vi "SpamDigit_v13.vi"() -> ()   [LabVIEW 2015]
uses:
  <vilib>/Platform/TimedLoop/XDataNode/timing_clust.ctl
  <vilib>/Platform/TimedLoop/XDataNode/nitl_modes.ctl
  <vilib>/Platform/TimedLoop/XDataNode/wakeup.ctl
  <vilib>/Utility/inputDevices.llb/keyboardAcquire.vi
  <vilib>/Utility/file.llb/Write To Spreadsheet File (string).vi
  <vilib>/Platform/TimedLoop/XDataNode/XDataNode.xnode
  <vilib>/Platform/TimedLoop/XDataNode/XDNodeRunTimeDep.lvlib
panel:
  out "Spam 2":i32
  out "seg":bool
  out "prim":bool
  out "tempo_rel":dbl[](array[numeric])
  out "erro":dbl[](array[numeric])
  out "total":dbl[](array[numeric])
  in  "Tab Control":enum32{"Config", "Exec"}(tab)
  in  "msg_inver":string="Na tela irão aparecer uma sequência de números. Após a sequência a mensagem \"comece!\" aparecerá e imediatamente você deve digitar os números na ordem inversas que eles apareceram. A quantidade de números irá aumentar gradualmente.                                           Pressione a tecla \"0\" para iniciar!"
  in  "Spam_1_I":string="24"
  in  "Spam_2_I":string="415" caption="Spam_2"
  in  "Spam_1_2_I":string="57"
  in  "Spam_2_2_I":string="629"
  in  "Spam_3_I":string="3272" caption="Spam_2"
  in  "Spam_4_I":string="15286" caption="Spam_2"
  in  "Spam_5_I":string="539418" caption="Spam_2"
  in  "Spam_6_I":string="8129365" caption="Spam_2"
  in  "Spam_7_I":string="72819653" caption="Spam_2"
  in  "Spam_8_I":string="591742817" caption="Spam_2"
  in  "Spam_9_I":string="4273164395" caption="Spam_2"
  in  "Spam_3_2_I":string="4968"
  in  "Spam_4_2_I":string="61843"
  in  "Spam_5_3_I":string="724856"
  in  "Spam_6_2_I":string="4739128"
  in  "Spam_7_2_I":string="94376258"
  in  "Spam_8_2_I":string="417938663"
  in  "Spam_9_2_I":string="7583672861"
  in  "Spam_1":string="17"
  in  "N_max spam":i32=9
  in  "Spam_2":string="582"
  in  "Spam_1_2":string="63"
  in  "Spam_2_2":string="694"
  in  "sensib":i32=200
  in  "Tempo1":u32=500
  in  "Tempo_2":u32=500
  in  "Spam_3":string="6439" caption="Spam_2"
  in  "Spam_4":string="42731" caption="Spam_2"
  in  "Spam_5":string="619473" caption="Spam_2"
  in  "Spam_6":string="5917428" caption="Spam_2"
  in  "Spam_7":string="38295174" caption="Spam_2"
  in  "Spam_8":string="275862584" caption="Spam_2"
  in  "Spam_9":string="4739128415" caption="Spam_2"
  in  "Spam_3_2":string="7286"
  in  "Spam_4_2":string="75836"
  in  "Spam_5_2":string="619473"
  in  "Spam_6_2":string="4179386"
  in  "Spam_7_2":string="58192647"
  in  "Spam_8_2":string="713942568"
  in  "Spam_9_2":string="8129365629"
  in  "comece":i32=300
  in  "aguarde":i32=1000
  in  "msg_direto":string=" Na tela irão aparecer uma sequência de números. Após a sequência a mensagem \"comece!\" aparecerá e imediatamente você deve digitar os números na mesma ordem que eles apareceram. A quantidade de números irá aumentar gradualmente.                                            Pressione a tecla \"0\" para iniciar!"
  in  "direto":bool
  in  "inver":bool
  in  "ambos":bool
  in  "print":string
  out "Aguarde":string
  in  "iniciar":bool
  out "Comece":string
  out "msg":string
  out "array2":T1(array[ring])
  in  "Spam":string="123"
  out "cont_erro":dbl
  out "error":dbl[](array[numeric])
  out "time":i32[](array[numeric])
  out "size":i32
  out "array":string[](array[string])
  # "Inverso"
  # "Direto"
  # "Número máx. spam"
  # "Tentativas"
  # "Spam"
  # "Spam"
  # "Tentativas"
  # "1"
  # "1"
  # "Sensibilidade (ms)"
  # "2"
  # "2"
  # "3"
  # "Duração do número (ms)"
  # "3"
  # "4"
  # "4"
  # "Intervalo entre os números (ms)"
  # "5"
  # "5"
  # "6"
  # "Duração do comece (ms)"
  # "6"
  # "7"
  # "7"
  # "8"
  # "Intervalo entre as tentativas (ms)"
  # "8"
  # "9"
  # "9"
  # "Só direto?"
  # "Mensagem inicial"
  # "Mensagem inicial"
  # "Só inverso?"
  # "Ambos"
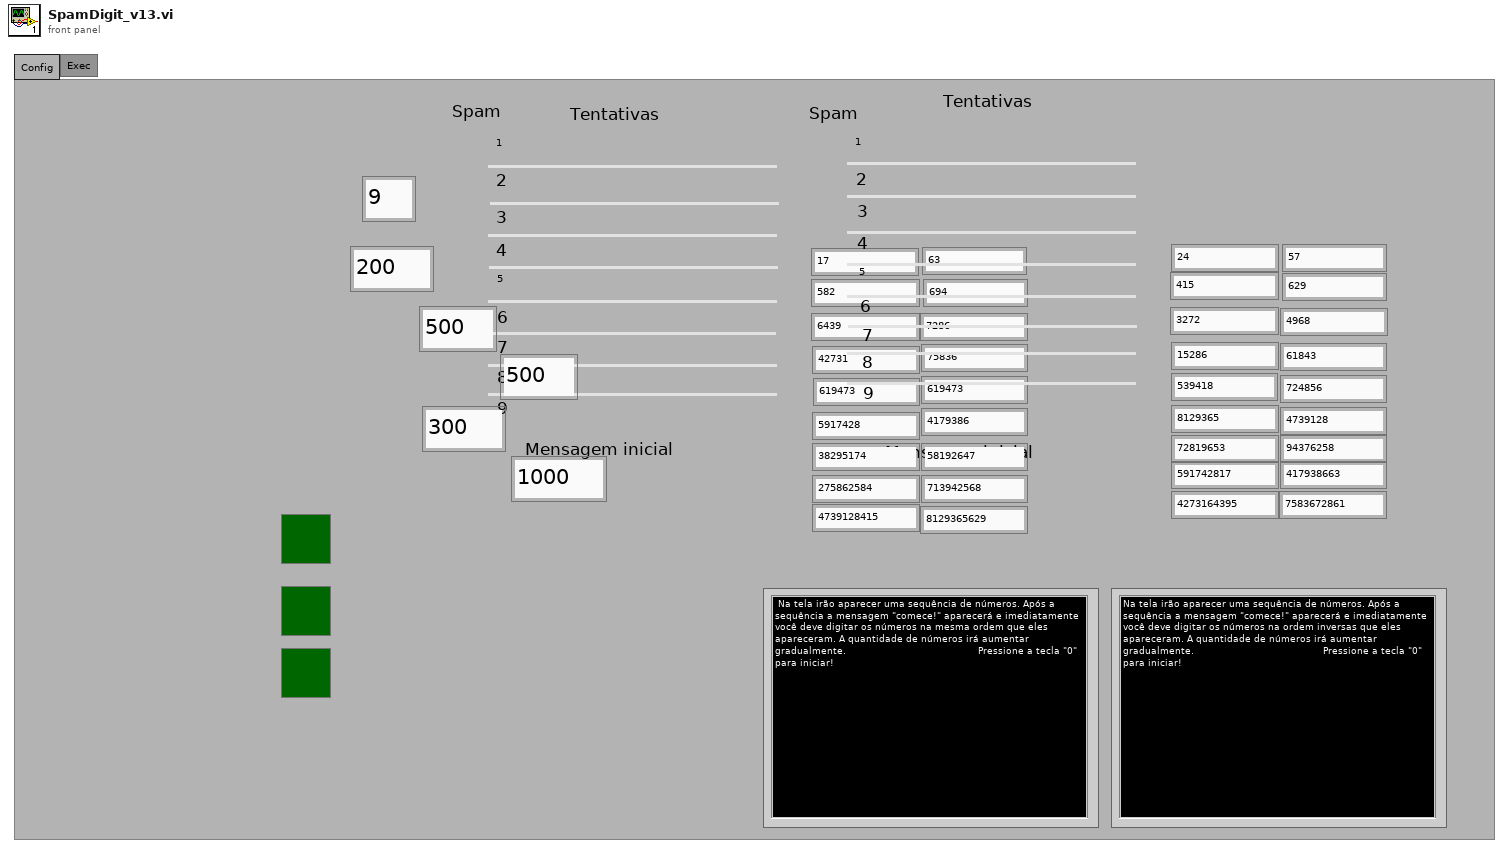
[diagram p1: front panel]
types:
  T1 = enum16{"0", "1", "2", "3", "4", "5", "6", "7", "8", "9", "A", "B", "C", "D", "E", "F", "G", "H", "I", "J", "K", "L", "M", "N", "O", "P", "Q", "R", "S", "T", "U", "V", "W", "X", "Y", "Z", "F1", "F2", "F3", "F4", "F5", "F6", "F7", "F8", "F9", "F10", "F11", "F12", "F13", "F14", "F15", "ADD", "BACK", "BACKSLASH", "CAPITAL", "COMMA", "DECIMAL", "DELETE", "DIVIDE", "DOWN", "END", "EQUALS", "ESCAPE", "GRAVE (`)", "HOME", "INSERT", "LBRACKET", "LCONTROL", "LEFT", "L ALT", "LSHIFT", "LWIN", "MINUS", "MULTIPLY", "NEXT", "NUMLOCK", "NUMPAD_0", "NUMPAD_1", "NUMPAD_2", "NUMPAD_3", "NUMPAD_4", "NUMPAD_5", "NUMPAD_6", "NUMPAD_7", "NUMPAD_8", "NUMPAD_9", "PAUSE", "PERIOD", "PRIOR (PG UP)", "RBRACKET", "RCONTROL", "RETURN", "RIGHT", "R ALT", "RSHIFT", "RWIN", "SCROLL", "SEMICOLON", "SLASH", "SPACE", "SUBTRACT", "TAB", "UP", "ENTER (num pad)", "' (quote)"}[]
  T2 = typedef "XDNodeRunTimeDep.lvlib/timing_clust.ctl" = cluster{"Expected End [f-1]":u64, "Actual End [f-1]":u64, "Finished Late? [f-1]":bool, "Expected End [i-1]":u64, "Actual End [i-1]":u64, "Finished Late? [i-1]":bool, "Expected Start [i]":u64, "Actual Start [i]":u64, "Expected Start [f]":u64, "Actual Start [f]":u64, "Source Name":string, "Structure Name":string, "Period":i64, "Deadline":i64, "Offset":i64, "Start":i64, "Priority":i32, "Timeout":i32, "Mode":T3, "Wakeup Reason":T4, "Error":errorcluster, "Source Type":string, "Secondary Source Type":string, "Global End Time":u64, "Global Start Time":u64, "Frame Duration":u64, "Iteration Duration":u64, "Assigned CPU":i32, "I/O Scan Engine Mode":u32}
  T3 = typedef "XDNodeRunTimeDep.lvlib/nitl_modes.ctl" = enum32{"No Change", "Process missed periods, maintain original phase", "Discard missed periods, maintain original phase", "Process missed periods, ignore original phase", "Discard missed periods, ignore original phase"}
  T4 = typedef "XDNodeRunTimeDep.lvlib/wakeup.ctl" = enum32{"Normal", "Aborted", "Asynchronous wakeup", "Timing source error", "Timed loop error", "Timeout"}
  T5 = enum16{"0", "1", "2", "3", "4", "5", "6", "7", "8", "9", "A", "B", "C", "D", "E", "F", "G", "H", "I", "J", "K", "L", "M", "N", "O", "P", "Q", "R", "S", "T", "U", "V", "W", "X", "Y", "Z", "F1", "F2", "F3", "F4", "F5", "F6", "F7", "F8", "F9", "F10", "F11", "F12", "F13", "F14", "F15", "ADD", "BACK", "BACKSLASH", "CAPITAL", "COMMA", "DECIMAL", "DELETE", "DIVIDE", "DOWN", "END", "EQUALS", "ESCAPE", "GRAVE (`)", "HOME", "INSERT", "LBRACKET", "LCONTROL", "LEFT", "L ALT", "LSHIFT", "LWIN", "MINUS", "MULTIPLY", "NEXT", "NUMLOCK", "NUMPAD_0", "NUMPAD_1", "NUMPAD_2", "NUMPAD_3", "NUMPAD_4", "NUMPAD_5", "NUMPAD_6", "NUMPAD_7", "NUMPAD_8", "NUMPAD_9", "PAUSE", "PERIOD", "PRIOR (PG UP)", "RBRACKET", "RCONTROL", "RETURN", "RIGHT", "R ALT", "RSHIFT", "RWIN", "SCROLL", "SEMICOLON", "SLASH", "SPACE", "SUBTRACT", "TAB", "UP", "ENTER (num pad)", "' (quote)"}
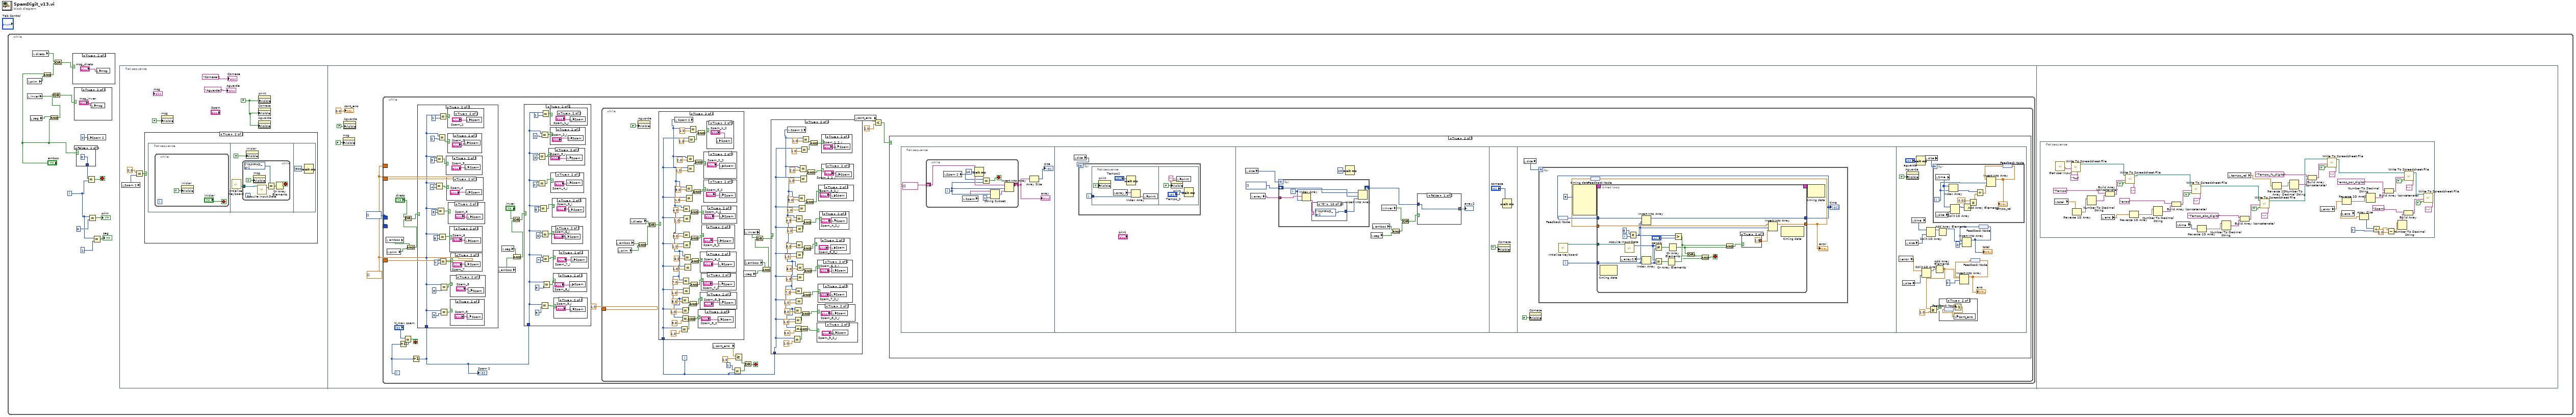
[diagram p0: block diagram]
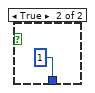
[diagram p4: hidden frame]
diagram:
  n1 = while {
    i -> [w11]
    stop <- w15 stop-if-true
    n2 = local read "prim"() -> (w4:bool)
    n3 = local read "inver"() -> (w7:bool)
    n4 = local read "seg"() -> (w3:bool)
    n5 = local read "direto"() -> (w9:bool)
    n6 = And(x="ambos", y=w4) -> (x .and. y?=w5:bool)
    n7 = And(x=w3, y="ambos") -> (x .and. y?=w1:bool)
    n8 = Or(x=w7, y=w1) -> (x .or. y?=w6:bool)
    n9 = Or(x=w9, y=w5) -> (x .or. y?=w8:bool)
    n10 = case shown="True" w8 {
      frame False {
      }
      frame True {
        n11 = local write "msg"("msg_direto") -> ()
      }
    }
    n12 = case shown="True" w6 {
      frame False {
      }
      frame True {
        n13 = local write "msg"("msg_inver") -> ()
      }
    }
    n14 = case shown="False" "ambos" {
      tunnel: [0 1] -> w16
      frame False {
      }
      frame True {
      }
    }
    n15 = Equal?(x=w16, y=w11) -> (x = y?=w15:bool)
    n16 = local write "Spam 2"(0 ("Spam 2")) -> ()
    n17 = Equal?(x=w11, y=0) -> (x = y?=→"prim":bool)
    n18 = Equal?(x=w11, y=1) -> (x = y?=→"seg":bool)
    n19 = flat-sequence {
      frame #0 {
        w23 = FALSE ("Visible")
        n20 = local read "Spam 2"() -> (w26:i32)
        n21 = Equal?(x=0.0, y=w26) -> (x = y?=w27:bool)
        n22 = case shown="True" w27 {
          frame False {
          }
          frame True {
            n23 = flat-sequence {
              frame #0 {
                n24 = while {
                  stop <- "iniciar" stop-if-true
                  n25 = property on="iniciar" class="Bool"("Visible"=TRUE) -> ()  [unwired: 2 in, 2 out]
                }
              }
              frame #1 {
                n26 = call <vilib>:"Intialize Keyboard.vi"() -> ("device ID"=w31:refnum<k1>)  [unwired: 10 in, 1 out]
                n27 = while {
                  tunnel: w31 -> [w37]
                  stop <- w33 stop-if-true
                  w35 = T1 [enum."NUMPAD_0"] items=["0", "1", "2", "3", "4", "5", "6", "7", "8", "9", "A", "B", "C", "D", "E", "F", "G", "H", "I", "J", "K", "L", "M", "N", "O", "P", "Q", "R", "S", "T", "U", "V", "W", "X", "Y", "Z", "F1", "F2", "F3", "F4", "F5", "F6", "F7", "F8", "F9", "F10", "F11", "F12", "F13", "F14", "F15", "ADD", "BACK", "BACKSLASH", "CAPITAL", "COMMA", "DECIMAL", "DELETE", "DIVIDE", "DOWN", "END", "EQUALS", "ESCAPE", "GRAVE (`)", "HOME", "INSERT", "LBRACKET", "LCONTROL", "LEFT", "L ALT", "LSHIFT", "LWIN", "MINUS", "MULTIPLY", "NEXT", "NUMLOCK", "NUMPAD_0", "NUMPAD_1", "NUMPAD_2", "NUMPAD_3", "NUMPAD_4", "NUMPAD_5", "NUMPAD_6", "NUMPAD_7", "NUMPAD_8", "NUMPAD_9", "PAUSE", "PERIOD", "PRIOR (PG UP)", "RBRACKET", "RCONTROL", "RETURN", "RIGHT", "R ALT", "RSHIFT", "RWIN", "SCROLL", "SEMICOLON", "SLASH", "SPACE", "SUBTRACT", "TAB", "UP", "ENTER (num pad)", "' (quote)"] ("x")
                  n28 = property on="msg" class="Str"("Visible"=TRUE) -> ()  [unwired: 2 in, 2 out]
                  n29 = call-poly <vilib>:"Acquire Input Data.vi"("device ID"=w37) -> ("keys pressed"=w36:T1)  [unwired: 16 in, 2 out]
                  n30 = Equal?(x=w35, y=w36) -> (x = y?=w34:bool[])
                  n31 = Or Array Elements(Boolean array=w34) -> (logical OR=w33:bool)
                }
                n32 = property on="iniciar" class="Bool"("Visible"=FALSE) -> ()  [unwired: 2 in, 2 out]
              }
              frame #2 {
                n33 = Wait (ms)(milliseconds to wait=u32 500) -> ()  [unwired: 1 out]
              }
            }
          }
        }
        n34 = property on="msg" class="Str"("Visible"=FALSE) -> ()  [unwired: 2 in, 2 out]
        n35 = property on="Comece" class="Str"("Visible"=w23) -> ()  [unwired: 2 in, 2 out]
        n36 = property on="Aguarde" class="Str"("Visible"=w23) -> ()  [unwired: 2 in, 2 out]
        n37 = property on="print" class="Str"("Visible"=w23) -> ()  [unwired: 2 in, 2 out]
        "Aguarde" <- "Aguarde!" ("Caixa de texto 2")
        "Comece" <- "Comece!" ("Caixa de texto 2")
      }
      frame #1 {
        w40 = dbl[] []
        w42 = i32[] []
        n38 = property on="msg" class="Str"("Visible"=FALSE) -> ()  [unwired: 2 in, 2 out]
        n39 = property on="Aguarde" class="Str"("Visible"=FALSE) -> ()  [unwired: 2 in, 2 out]
        n40 = while {
          border: w42 -> [_]
          border: w40 -> [_]
          border: w42 -> [_]
          border: w40 -> [_]
          border: w40 -> [_]
          i -> [w58]
          stop <- w59 stop-if-true
          n41 = local read "ambos"() -> (w50:bool)
          n42 = local read "prim"() -> (w49:bool)
          n43 = Increment(x=w58) -> (x+1=w60:i32)
          n44 = Equal?(x="N_max spam", y=w60) -> (x = y?=w59:bool)
          n45 = And(x=w50, y=w49) -> (x .and. y?=w48:bool)
          n46 = Or(x="direto", y=w48) -> (x .or. y?=w53:bool)
          n47 = Increment(x=w58) -> (x+1=w55:i32)
          "Spam 2" <- w55
          n48 = case shown="True" w53 {
            tunnel: w55 -> [_ w90]
            frame False {
            }
            frame True {
              n49 = Equal?(x=w90, y=4) -> (x = y?=w101:bool)
              n50 = Equal?(x=w90, y=3) -> (x = y?=w102:bool)
              n51 = Equal?(x=w90, y=5) -> (x = y?=w98:bool)
              n52 = Equal?(x=w90, y=2) -> (x = y?=w105:bool)
              n53 = Equal?(x=w90, y=6) -> (x = y?=w96:bool)
              n54 = Equal?(x=w90, y=1) -> (x = y?=w107:bool)
              n55 = Equal?(x=w90, y=7) -> (x = y?=w94:bool)
              n56 = Equal?(x=w90, y=8) -> (x = y?=w92:bool)
              n57 = Equal?(x=w90, y=9) -> (x = y?=w89:bool)
              n58 = case shown="True" w102 {
                frame False {
                }
                frame True {
                  n59 = local write "Spam"("Spam_3") -> ()
                }
              }
              n60 = case shown="True" w101 {
                frame False {
                }
                frame True {
                  n61 = local write "Spam"("Spam_4") -> ()
                }
              }
              n62 = case shown="True" w107 {
                frame False {
                }
                frame True {
                  n63 = local write "Spam"("Spam_1") -> ()
                }
              }
              n64 = case shown="True" w105 {
                frame False {
                }
                frame True {
                  n65 = local write "Spam"("Spam_2") -> ()
                }
              }
              n66 = case shown="True" w98 {
                frame False {
                }
                frame True {
                  n67 = local write "Spam"("Spam_5") -> ()
                }
              }
              n68 = case shown="True" w96 {
                frame False {
                }
                frame True {
                  n69 = local write "Spam"("Spam_6") -> ()
                }
              }
              n70 = case shown="True" w92 {
                frame False {
                }
                frame True {
                  n71 = local write "Spam"("Spam_8") -> ()
                }
              }
              n72 = case shown="True" w89 {
                frame False {
                }
                frame True {
                  n73 = local write "Spam"("Spam_9") -> ()
                }
              }
              n74 = case shown="True" w94 {
                frame False {
                }
                frame True {
                  n75 = local write "Spam"("Spam_7") -> ()
                }
              }
            }
          }
          n76 = local read "ambos"() -> (w47:bool)
          n77 = local read "seg"() -> (w46:bool)
          n78 = And(x=w46, y=w47) -> (x .and. y?=w45:bool)
          n79 = Or(x="inver", y=w45) -> (x .or. y?=w51:bool)
          n80 = case shown="True" w51 {
            tunnel: w55 -> [_ w70]
            frame False {
            }
            frame True {
              n81 = Equal?(x=w70, y=4) -> (x = y?=w66:bool)
              n82 = Equal?(x=w70, y=3) -> (x = y?=w67:bool)
              n83 = Equal?(x=w70, y=5) -> (x = y?=w65:bool)
              n84 = Equal?(x=w70, y=2) -> (x = y?=w68:bool)
              n85 = Equal?(x=w70, y=9) -> (x = y?=w61:bool)
              n86 = Equal?(x=w70, y=6) -> (x = y?=w64:bool)
              n87 = Equal?(x=w70, y=1) -> (x = y?=w69:bool)
              n88 = Equal?(x=w70, y=7) -> (x = y?=w63:bool)
              n89 = Equal?(x=w70, y=8) -> (x = y?=w62:bool)
              n90 = case shown="True" w67 {
                frame False {
                }
                frame True {
                  n91 = local write "Spam"("Spam_3_I") -> ()
                }
              }
              n92 = case shown="True" w69 {
                frame False {
                }
                frame True {
                  n93 = local write "Spam"("Spam_1_I") -> ()
                }
              }
              n94 = case shown="True" w68 {
                frame False {
                }
                frame True {
                  n95 = local write "Spam"("Spam_2_I") -> ()
                }
              }
              n96 = case shown="True" w66 {
                frame False {
                }
                frame True {
                  n97 = local write "Spam"("Spam_4_I") -> ()
                }
              }
              n98 = case shown="True" w64 {
                frame False {
                }
                frame True {
                  n99 = local write "Spam"("Spam_6_I") -> ()
                }
              }
              n100 = case shown="True" w65 {
                frame False {
                }
                frame True {
                  n101 = local write "Spam"("Spam_5_I") -> ()
                }
              }
              n102 = case shown="True" w63 {
                frame False {
                }
                frame True {
                  n103 = local write "Spam"("Spam_7_I") -> ()
                }
              }
              n104 = case shown="True" w62 {
                frame False {
                }
                frame True {
                  n105 = local write "Spam"("Spam_8_I") -> ()
                }
              }
              n106 = case shown="True" w61 {
                frame False {
                }
                frame True {
                  n107 = local write "Spam"("Spam_9_I") -> ()
                }
              }
            }
          }
          n108 = while {
            border: 1.0 -> [_]
            i -> [w127]
            stop <- w132 stop-if-true
            n109 = local read "ambos"() -> (w121:bool)
            n110 = local read "prim"() -> (w122:bool)
            n111 = local read "direto"() -> (w125:bool)
            n112 = And(x=w121, y=w122) -> (x .and. y?=w120:bool)
            n113 = property on="Aguarde" class="Str"("Visible"=FALSE) -> ()  [unwired: 2 in, 2 out]
            n114 = Or(x=w125, y=w120) -> (x .or. y?=w126:bool)
            n115 = case shown="True" w126 {
              tunnel: w127 -> [_ w196]
              frame False {
              }
              frame True {
                n116 = local read "Spam 2"() -> (w194:i32)
                n117 = Equal?(x=w196, y=1.0) -> (x = y?=w197:bool)
                n118 = Equal?(x=w194, y=8.0) -> (x = y?=w203:bool)
                n119 = Equal?(x=w196, y=1.0) -> (x = y?=w202:bool)
                n120 = Equal?(x=w194, y=9.0) -> (x = y?=w198:bool)
                n121 = Equal?(x=w194, y=7.0) -> (x = y?=w208:bool)
                n122 = Equal?(x=w196, y=1.0) -> (x = y?=w207:bool)
                n123 = Equal?(x=w194, y=4.0) -> (x = y?=w223:bool)
                n124 = Equal?(x=w194, y=5.0) -> (x = y?=w218:bool)
                n125 = Equal?(x=w196, y=1.0) -> (x = y?=w222:bool)
                n126 = Equal?(x=w196, y=1.0) -> (x = y?=w217:bool)
                n127 = Equal?(x=w194, y=6.0) -> (x = y?=w213:bool)
                n128 = Equal?(x=w196, y=1.0) -> (x = y?=w212:bool)
                n129 = Equal?(x=w194, y=3.0) -> (x = y?=w228:bool)
                n130 = Equal?(x=w196, y=1.0) -> (x = y?=w227:bool)
                n131 = Equal?(x=w194, y=2.0) -> (x = y?=w233:bool)
                n132 = Equal?(x=w196, y=1.0) -> (x = y?=w232:bool)
                n133 = Equal?(x=w196, y=1.0) -> (x = y?=w237:bool)
                n134 = And(x=w198, y=w197) -> (x .and. y?=w195:bool)
                n135 = Equal?(x=w194, y=1.0) -> (x = y?=w238:bool)
                n136 = And(x=w203, y=w202) -> (x .and. y?=w201:bool)
                n137 = And(x=w208, y=w207) -> (x .and. y?=w206:bool)
                n138 = And(x=w223, y=w222) -> (x .and. y?=w221:bool)
                n139 = And(x=w218, y=w217) -> (x .and. y?=w216:bool)
                n140 = And(x=w213, y=w212) -> (x .and. y?=w211:bool)
                n141 = And(x=w228, y=w227) -> (x .and. y?=w226:bool)
                n142 = And(x=w233, y=w232) -> (x .and. y?=w231:bool)
                n143 = And(x=w238, y=w237) -> (x .and. y?=w236:bool)
                n144 = case shown="True" w195 {
                  frame False {
                  }
                  frame True {
                    n145 = local write "Spam"("Spam_9_2") -> ()
                  }
                }
                n146 = case shown="True" w201 {
                  frame False {
                  }
                  frame True {
                    n147 = local write "Spam"("Spam_8_2") -> ()
                  }
                }
                n148 = case shown="True" w211 {
                  frame False {
                  }
                  frame True {
                    n149 = local write "Spam"("Spam_6_2") -> ()
                  }
                }
                n150 = case shown="True" w206 {
                  frame False {
                  }
                  frame True {
                    n151 = local write "Spam"("Spam_7_2") -> ()
                  }
                }
                n152 = case shown="True" w221 {
                  frame False {
                  }
                  frame True {
                    n153 = local write "Spam"("Spam_4_2") -> ()
                  }
                }
                n154 = case shown="True" w216 {
                  frame False {
                  }
                  frame True {
                    n155 = local write "Spam"("Spam_5_2") -> ()
                  }
                }
                n156 = case shown="True" w231 {
                  frame False {
                  }
                  frame True {
                    n157 = local write "Spam"("Spam_2_2") -> ()
                  }
                }
                n158 = case shown="True" w226 {
                  frame False {
                  }
                  frame True {
                    n159 = local write "Spam"("Spam_3_2") -> ()
                  }
                }
                n160 = case shown="True" w236 {
                  frame False {
                  }
                  frame True {
                    n161 = local write "Spam"("Spam_1_2") -> ()
                  }
                }
              }
            }
            n162 = local read "cont_erro"() -> (w137:dbl)
            n163 = Equal?(x=1, y=w127) -> (x = y?=w134:bool)
            n164 = Greater Or Equal?(x=w137, y=2.0) -> (x >= y?=w133:bool)
            n165 = local read "seg"() -> (w119:bool)
            n166 = Or(x=w133, y=w134) -> (x .or. y?=w132:bool)
            n167 = local read "inver"() -> (w124:bool)
            n168 = local read "ambos"() -> (w118:bool)
            n169 = And(x=w118, y=w119) -> (x .and. y?=w117:bool)
            n170 = Or(x=w124, y=w117) -> (x .or. y?=w123:bool)
            n171 = case shown="True" w123 {
              tunnel: w127 -> [_ w148]
              frame False {
              }
              frame True {
                n172 = local read "Spam 2"() -> (w149:i32)
                n173 = Equal?(x=w148, y=1.0) -> (x = y?=w150:bool)
                n174 = Equal?(x=w149, y=8.0) -> (x = y?=w155:bool)
                n175 = Equal?(x=w148, y=1.0) -> (x = y?=w154:bool)
                n176 = Equal?(x=w149, y=9.0) -> (x = y?=w151:bool)
                n177 = Equal?(x=w149, y=7.0) -> (x = y?=w159:bool)
                n178 = Equal?(x=w148, y=1.0) -> (x = y?=w158:bool)
                n179 = Equal?(x=w149, y=4.0) -> (x = y?=w171:bool)
                n180 = Equal?(x=w149, y=5.0) -> (x = y?=w167:bool)
                n181 = Equal?(x=w148, y=1.0) -> (x = y?=w170:bool)
                n182 = Equal?(x=w148, y=1.0) -> (x = y?=w166:bool)
                n183 = Equal?(x=w149, y=6.0) -> (x = y?=w163:bool)
                n184 = Equal?(x=w148, y=1.0) -> (x = y?=w162:bool)
                n185 = Equal?(x=w149, y=3.0) -> (x = y?=w175:bool)
                n186 = Equal?(x=w148, y=1.0) -> (x = y?=w174:bool)
                n187 = Equal?(x=w149, y=2.0) -> (x = y?=w179:bool)
                n188 = Equal?(x=w148, y=1.0) -> (x = y?=w178:bool)
                n189 = Equal?(x=w148, y=1.0) -> (x = y?=w147:bool)
                n190 = And(x=w151, y=w150) -> (x .and. y?=w138:bool)
                n191 = Equal?(x=w149, y=1.0) -> (x = y?=w182:bool)
                n192 = And(x=w155, y=w154) -> (x .and. y?=w139:bool)
                n193 = And(x=w159, y=w158) -> (x .and. y?=w140:bool)
                n194 = And(x=w171, y=w170) -> (x .and. y?=w143:bool)
                n195 = And(x=w167, y=w166) -> (x .and. y?=w142:bool)
                n196 = And(x=w163, y=w162) -> (x .and. y?=w141:bool)
                n197 = And(x=w175, y=w174) -> (x .and. y?=w144:bool)
                n198 = And(x=w179, y=w178) -> (x .and. y?=w145:bool)
                n199 = And(x=w182, y=w147) -> (x .and. y?=w146:bool)
                n200 = case shown="True" w142 {
                  frame False {
                  }
                  frame True {
                    n201 = local write "Spam"("Spam_5_3_I") -> ()
                  }
                }
                n202 = case shown="True" w138 {
                  frame False {
                  }
                  frame True {
                    n203 = local write "Spam"("Spam_9_2_I") -> ()
                  }
                }
                n204 = case shown="True" w141 {
                  frame False {
                  }
                  frame True {
                    n205 = local write "Spam"("Spam_6_2_I") -> ()
                  }
                }
                n206 = case shown="True" w139 {
                  frame False {
                  }
                  frame True {
                    n207 = local write "Spam"("Spam_8_2_I") -> ()
                  }
                }
                n208 = case shown="True" w140 {
                  frame False {
                  }
                  frame True {
                    n209 = local write "Spam"("Spam_7_2_I") -> ()
                  }
                }
                n210 = case shown="True" w144 {
                  frame False {
                  }
                  frame True {
                    n211 = local write "Spam"("Spam_3_2_I") -> ()
                  }
                }
                n212 = case shown="True" w143 {
                  frame False {
                  }
                  frame True {
                    n213 = local write "Spam"("Spam_4_2_I") -> ()
                  }
                }
                n214 = case shown="True" w146 {
                  frame False {
                  }
                  frame True {
                    n215 = local write "Spam"("Spam_1_2_I") -> ()
                  }
                }
                n216 = case shown="True" w145 {
                  frame False {
                  }
                  frame True {
                    n217 = local write "Spam"("Spam_2_2_I") -> ()
                  }
                }
              }
            }
            n218 = local read "cont_erro"() -> (w129:dbl)
            n219 = Less?(x=w129, y=2.0) -> (x < y?=w130:bool)
            n220 = case shown="True" w130 {
              frame False {
              }
              frame True {
                n221 = flat-sequence {
                  frame #0 {
                    n222 = while {
                      shift-right: [w257] -> w251
                      shift-left: string[] [] -> [w261]
                      i -> [w258]
                      stop <- w253 stop-if-true
                      n223 = local read "Spam 2"() -> (w254:i32)
                      n224 = local read "Spam"() -> (w255:string)
                      n225 = Wait (ms)(milliseconds to wait=u32 10) -> ()  [unwired: 1 out]
                      n226 = Equal?(x=w254, y=w258) -> (x = y?=w253:bool)
                      n227 = String Subset(string=w255, offset (0)=w258, length (rest)=1 ("length (rest)")) -> (substring=w256:string)
                      n228 = Insert Into Array(array=w261, index=w258, new element=w256) -> (w257:string[])
                    }
                    "array" <- w251
                    n229 = Array Size(array=w251) -> (size(s)=→"size":i32)
                  }
                  frame #1 {
                    n230 = local read "size"() -> (w262:i32)
                    n231 = for {
                      N: w262 -> [_]
                      i -> [w263]
                      n232 = flat-sequence {
                        tunnel: w263 -> [w266]
                        frame #0 {
                          n233 = property on="print" class="Str"("Visible"=TRUE) -> ()  [unwired: 2 in, 2 out]
                          n234 = local read "array"() -> (w268:string[])
                          n235 = Wait (ms)(milliseconds to wait="Tempo1") -> ()  [unwired: 1 out]
                          n236 = Index Array(array=w268, index=w266) -> (element=w267:string)
                          n237 = local write "print"(w267) -> ()
                        }
                        frame #1 {
                          n238 = property on="print" class="Str"("Visible"=FALSE) -> ()  [unwired: 2 in, 2 out]
                          n239 = local write "print"("" ("String")) -> ()
                          n240 = Wait (ms)(milliseconds to wait="Tempo_2") -> ()  [unwired: 1 out]
                        }
                      }
                    }
                  }
                  frame #2 {
                    w280 = T1 [] items=["0", "1", "2", "3", "4", "5", "6", "7", "8", "9", "A", "B", "C", "D", "E", "F", "G", "H", "I", "J", "K", "L", "M", "N", "O", "P", "Q", "R", "S", "T", "U", "V", "W", "X", "Y", "Z", "F1", "F2", "F3", "F4", "F5", "F6", "F7", "F8", "F9", "F10", "F11", "F12", "F13", "F14", "F15", "ADD", "BACK", "BACKSLASH", "CAPITAL", "COMMA", "DECIMAL", "DELETE", "DIVIDE", "DOWN", "END", "EQUALS", "ESCAPE", "GRAVE (`)", "HOME", "INSERT", "LBRACKET", "LCONTROL", "LEFT", "L ALT", "LSHIFT", "LWIN", "MINUS", "MULTIPLY", "NEXT", "NUMLOCK", "NUMPAD_0", "NUMPAD_1", "NUMPAD_2", "NUMPAD_3", "NUMPAD_4", "NUMPAD_5", "NUMPAD_6", "NUMPAD_7", "NUMPAD_8", "NUMPAD_9", "PAUSE", "PERIOD", "PRIOR (PG UP)", "RBRACKET", "RCONTROL", "RETURN", "RIGHT", "R ALT", "RSHIFT", "RWIN", "SCROLL", "SEMICOLON", "SLASH", "SPACE", "SUBTRACT", "TAB", "UP", "ENTER (num pad)", "' (quote)"]
                    n241 = local read "size"() -> (w282:i32)
                    n242 = local read "array"() -> (w281:string[])
                    n243 = for {
                      N: w282 -> [_]
                      tunnel: w281 -> [w291]
                      shift-right: [w287] -> w277
                      shift-left: w280 -> [w286]
                      i -> [w288]
                      n244 = Index Array(array=w291, index=w288) -> (element=w290:string)
                      n245 = case shown="\"9\"" w290 {
                        tunnel: [w292 w293 w294 w295 w296 w297 w298 w299 w300 w301] -> w289
                        frame "0", Default {
                          w292 = T1 [enum."NUMPAD_0"] items=["0", "1", "2", "3", "4", "5", "6", "7", "8", "9", "A", "B", "C", "D", "E", "F", "G", "H", "I", "J", "K", "L", "M", "N", "O", "P", "Q", "R", "S", "T", "U", "V", "W", "X", "Y", "Z", "F1", "F2", "F3", "F4", "F5", "F6", "F7", "F8", "F9", "F10", "F11", "F12", "F13", "F14", "F15", "ADD", "BACK", "BACKSLASH", "CAPITAL", "COMMA", "DECIMAL", "DELETE", "DIVIDE", "DOWN", "END", "EQUALS", "ESCAPE", "GRAVE (`)", "HOME", "INSERT", "LBRACKET", "LCONTROL", "LEFT", "L ALT", "LSHIFT", "LWIN", "MINUS", "MULTIPLY", "NEXT", "NUMLOCK", "NUMPAD_0", "NUMPAD_1", "NUMPAD_2", "NUMPAD_3", "NUMPAD_4", "NUMPAD_5", "NUMPAD_6", "NUMPAD_7", "NUMPAD_8", "NUMPAD_9", "PAUSE", "PERIOD", "PRIOR (PG UP)", "RBRACKET", "RCONTROL", "RETURN", "RIGHT", "R ALT", "RSHIFT", "RWIN", "SCROLL", "SEMICOLON", "SLASH", "SPACE", "SUBTRACT", "TAB", "UP", "ENTER (num pad)", "' (quote)"] ("keys pressed")
                        }
                        frame "1" {
                          w293 = T1 [enum."NUMPAD_1"] items=["0", "1", "2", "3", "4", "5", "6", "7", "8", "9", "A", "B", "C", "D", "E", "F", "G", "H", "I", "J", "K", "L", "M", "N", "O", "P", "Q", "R", "S", "T", "U", "V", "W", "X", "Y", "Z", "F1", "F2", "F3", "F4", "F5", "F6", "F7", "F8", "F9", "F10", "F11", "F12", "F13", "F14", "F15", "ADD", "BACK", "BACKSLASH", "CAPITAL", "COMMA", "DECIMAL", "DELETE", "DIVIDE", "DOWN", "END", "EQUALS", "ESCAPE", "GRAVE (`)", "HOME", "INSERT", "LBRACKET", "LCONTROL", "LEFT", "L ALT", "LSHIFT", "LWIN", "MINUS", "MULTIPLY", "NEXT", "NUMLOCK", "NUMPAD_0", "NUMPAD_1", "NUMPAD_2", "NUMPAD_3", "NUMPAD_4", "NUMPAD_5", "NUMPAD_6", "NUMPAD_7", "NUMPAD_8", "NUMPAD_9", "PAUSE", "PERIOD", "PRIOR (PG UP)", "RBRACKET", "RCONTROL", "RETURN", "RIGHT", "R ALT", "RSHIFT", "RWIN", "SCROLL", "SEMICOLON", "SLASH", "SPACE", "SUBTRACT", "TAB", "UP", "ENTER (num pad)", "' (quote)"] ("keys pressed")
                        }
                        frame "2" {
                          w294 = T1 [enum."NUMPAD_2"] items=["0", "1", "2", "3", "4", "5", "6", "7", "8", "9", "A", "B", "C", "D", "E", "F", "G", "H", "I", "J", "K", "L", "M", "N", "O", "P", "Q", "R", "S", "T", "U", "V", "W", "X", "Y", "Z", "F1", "F2", "F3", "F4", "F5", "F6", "F7", "F8", "F9", "F10", "F11", "F12", "F13", "F14", "F15", "ADD", "BACK", "BACKSLASH", "CAPITAL", "COMMA", "DECIMAL", "DELETE", "DIVIDE", "DOWN", "END", "EQUALS", "ESCAPE", "GRAVE (`)", "HOME", "INSERT", "LBRACKET", "LCONTROL", "LEFT", "L ALT", "LSHIFT", "LWIN", "MINUS", "MULTIPLY", "NEXT", "NUMLOCK", "NUMPAD_0", "NUMPAD_1", "NUMPAD_2", "NUMPAD_3", "NUMPAD_4", "NUMPAD_5", "NUMPAD_6", "NUMPAD_7", "NUMPAD_8", "NUMPAD_9", "PAUSE", "PERIOD", "PRIOR (PG UP)", "RBRACKET", "RCONTROL", "RETURN", "RIGHT", "R ALT", "RSHIFT", "RWIN", "SCROLL", "SEMICOLON", "SLASH", "SPACE", "SUBTRACT", "TAB", "UP", "ENTER (num pad)", "' (quote)"] ("keys pressed")
                        }
                        frame "3" {
                          w295 = T1 [enum."NUMPAD_3"] items=["0", "1", "2", "3", "4", "5", "6", "7", "8", "9", "A", "B", "C", "D", "E", "F", "G", "H", "I", "J", "K", "L", "M", "N", "O", "P", "Q", "R", "S", "T", "U", "V", "W", "X", "Y", "Z", "F1", "F2", "F3", "F4", "F5", "F6", "F7", "F8", "F9", "F10", "F11", "F12", "F13", "F14", "F15", "ADD", "BACK", "BACKSLASH", "CAPITAL", "COMMA", "DECIMAL", "DELETE", "DIVIDE", "DOWN", "END", "EQUALS", "ESCAPE", "GRAVE (`)", "HOME", "INSERT", "LBRACKET", "LCONTROL", "LEFT", "L ALT", "LSHIFT", "LWIN", "MINUS", "MULTIPLY", "NEXT", "NUMLOCK", "NUMPAD_0", "NUMPAD_1", "NUMPAD_2", "NUMPAD_3", "NUMPAD_4", "NUMPAD_5", "NUMPAD_6", "NUMPAD_7", "NUMPAD_8", "NUMPAD_9", "PAUSE", "PERIOD", "PRIOR (PG UP)", "RBRACKET", "RCONTROL", "RETURN", "RIGHT", "R ALT", "RSHIFT", "RWIN", "SCROLL", "SEMICOLON", "SLASH", "SPACE", "SUBTRACT", "TAB", "UP", "ENTER (num pad)", "' (quote)"] ("keys pressed")
                        }
                        frame "4" {
                          w296 = T1 [enum."NUMPAD_4"] items=["0", "1", "2", "3", "4", "5", "6", "7", "8", "9", "A", "B", "C", "D", "E", "F", "G", "H", "I", "J", "K", "L", "M", "N", "O", "P", "Q", "R", "S", "T", "U", "V", "W", "X", "Y", "Z", "F1", "F2", "F3", "F4", "F5", "F6", "F7", "F8", "F9", "F10", "F11", "F12", "F13", "F14", "F15", "ADD", "BACK", "BACKSLASH", "CAPITAL", "COMMA", "DECIMAL", "DELETE", "DIVIDE", "DOWN", "END", "EQUALS", "ESCAPE", "GRAVE (`)", "HOME", "INSERT", "LBRACKET", "LCONTROL", "LEFT", "L ALT", "LSHIFT", "LWIN", "MINUS", "MULTIPLY", "NEXT", "NUMLOCK", "NUMPAD_0", "NUMPAD_1", "NUMPAD_2", "NUMPAD_3", "NUMPAD_4", "NUMPAD_5", "NUMPAD_6", "NUMPAD_7", "NUMPAD_8", "NUMPAD_9", "PAUSE", "PERIOD", "PRIOR (PG UP)", "RBRACKET", "RCONTROL", "RETURN", "RIGHT", "R ALT", "RSHIFT", "RWIN", "SCROLL", "SEMICOLON", "SLASH", "SPACE", "SUBTRACT", "TAB", "UP", "ENTER (num pad)", "' (quote)"] ("keys pressed")
                        }
                        frame "5" {
                          w297 = T1 [enum."NUMPAD_5"] items=["0", "1", "2", "3", "4", "5", "6", "7", "8", "9", "A", "B", "C", "D", "E", "F", "G", "H", "I", "J", "K", "L", "M", "N", "O", "P", "Q", "R", "S", "T", "U", "V", "W", "X", "Y", "Z", "F1", "F2", "F3", "F4", "F5", "F6", "F7", "F8", "F9", "F10", "F11", "F12", "F13", "F14", "F15", "ADD", "BACK", "BACKSLASH", "CAPITAL", "COMMA", "DECIMAL", "DELETE", "DIVIDE", "DOWN", "END", "EQUALS", "ESCAPE", "GRAVE (`)", "HOME", "INSERT", "LBRACKET", "LCONTROL", "LEFT", "L ALT", "LSHIFT", "LWIN", "MINUS", "MULTIPLY", "NEXT", "NUMLOCK", "NUMPAD_0", "NUMPAD_1", "NUMPAD_2", "NUMPAD_3", "NUMPAD_4", "NUMPAD_5", "NUMPAD_6", "NUMPAD_7", "NUMPAD_8", "NUMPAD_9", "PAUSE", "PERIOD", "PRIOR (PG UP)", "RBRACKET", "RCONTROL", "RETURN", "RIGHT", "R ALT", "RSHIFT", "RWIN", "SCROLL", "SEMICOLON", "SLASH", "SPACE", "SUBTRACT", "TAB", "UP", "ENTER (num pad)", "' (quote)"] ("keys pressed")
                        }
                        frame "6" {
                          w298 = T1 [enum."NUMPAD_6"] items=["0", "1", "2", "3", "4", "5", "6", "7", "8", "9", "A", "B", "C", "D", "E", "F", "G", "H", "I", "J", "K", "L", "M", "N", "O", "P", "Q", "R", "S", "T", "U", "V", "W", "X", "Y", "Z", "F1", "F2", "F3", "F4", "F5", "F6", "F7", "F8", "F9", "F10", "F11", "F12", "F13", "F14", "F15", "ADD", "BACK", "BACKSLASH", "CAPITAL", "COMMA", "DECIMAL", "DELETE", "DIVIDE", "DOWN", "END", "EQUALS", "ESCAPE", "GRAVE (`)", "HOME", "INSERT", "LBRACKET", "LCONTROL", "LEFT", "L ALT", "LSHIFT", "LWIN", "MINUS", "MULTIPLY", "NEXT", "NUMLOCK", "NUMPAD_0", "NUMPAD_1", "NUMPAD_2", "NUMPAD_3", "NUMPAD_4", "NUMPAD_5", "NUMPAD_6", "NUMPAD_7", "NUMPAD_8", "NUMPAD_9", "PAUSE", "PERIOD", "PRIOR (PG UP)", "RBRACKET", "RCONTROL", "RETURN", "RIGHT", "R ALT", "RSHIFT", "RWIN", "SCROLL", "SEMICOLON", "SLASH", "SPACE", "SUBTRACT", "TAB", "UP", "ENTER (num pad)", "' (quote)"] ("keys pressed")
                        }
                        frame "7" {
                          w299 = T1 [enum."NUMPAD_7"] items=["0", "1", "2", "3", "4", "5", "6", "7", "8", "9", "A", "B", "C", "D", "E", "F", "G", "H", "I", "J", "K", "L", "M", "N", "O", "P", "Q", "R", "S", "T", "U", "V", "W", "X", "Y", "Z", "F1", "F2", "F3", "F4", "F5", "F6", "F7", "F8", "F9", "F10", "F11", "F12", "F13", "F14", "F15", "ADD", "BACK", "BACKSLASH", "CAPITAL", "COMMA", "DECIMAL", "DELETE", "DIVIDE", "DOWN", "END", "EQUALS", "ESCAPE", "GRAVE (`)", "HOME", "INSERT", "LBRACKET", "LCONTROL", "LEFT", "L ALT", "LSHIFT", "LWIN", "MINUS", "MULTIPLY", "NEXT", "NUMLOCK", "NUMPAD_0", "NUMPAD_1", "NUMPAD_2", "NUMPAD_3", "NUMPAD_4", "NUMPAD_5", "NUMPAD_6", "NUMPAD_7", "NUMPAD_8", "NUMPAD_9", "PAUSE", "PERIOD", "PRIOR (PG UP)", "RBRACKET", "RCONTROL", "RETURN", "RIGHT", "R ALT", "RSHIFT", "RWIN", "SCROLL", "SEMICOLON", "SLASH", "SPACE", "SUBTRACT", "TAB", "UP", "ENTER (num pad)", "' (quote)"] ("keys pressed")
                        }
                        frame "8" {
                          w300 = T1 [enum."NUMPAD_8"] items=["0", "1", "2", "3", "4", "5", "6", "7", "8", "9", "A", "B", "C", "D", "E", "F", "G", "H", "I", "J", "K", "L", "M", "N", "O", "P", "Q", "R", "S", "T", "U", "V", "W", "X", "Y", "Z", "F1", "F2", "F3", "F4", "F5", "F6", "F7", "F8", "F9", "F10", "F11", "F12", "F13", "F14", "F15", "ADD", "BACK", "BACKSLASH", "CAPITAL", "COMMA", "DECIMAL", "DELETE", "DIVIDE", "DOWN", "END", "EQUALS", "ESCAPE", "GRAVE (`)", "HOME", "INSERT", "LBRACKET", "LCONTROL", "LEFT", "L ALT", "LSHIFT", "LWIN", "MINUS", "MULTIPLY", "NEXT", "NUMLOCK", "NUMPAD_0", "NUMPAD_1", "NUMPAD_2", "NUMPAD_3", "NUMPAD_4", "NUMPAD_5", "NUMPAD_6", "NUMPAD_7", "NUMPAD_8", "NUMPAD_9", "PAUSE", "PERIOD", "PRIOR (PG UP)", "RBRACKET", "RCONTROL", "RETURN", "RIGHT", "R ALT", "RSHIFT", "RWIN", "SCROLL", "SEMICOLON", "SLASH", "SPACE", "SUBTRACT", "TAB", "UP", "ENTER (num pad)", "' (quote)"] ("keys pressed")
                        }
                        frame "9" {
                          w301 = T1 [enum."NUMPAD_9"] items=["0", "1", "2", "3", "4", "5", "6", "7", "8", "9", "A", "B", "C", "D", "E", "F", "G", "H", "I", "J", "K", "L", "M", "N", "O", "P", "Q", "R", "S", "T", "U", "V", "W", "X", "Y", "Z", "F1", "F2", "F3", "F4", "F5", "F6", "F7", "F8", "F9", "F10", "F11", "F12", "F13", "F14", "F15", "ADD", "BACK", "BACKSLASH", "CAPITAL", "COMMA", "DECIMAL", "DELETE", "DIVIDE", "DOWN", "END", "EQUALS", "ESCAPE", "GRAVE (`)", "HOME", "INSERT", "LBRACKET", "LCONTROL", "LEFT", "L ALT", "LSHIFT", "LWIN", "MINUS", "MULTIPLY", "NEXT", "NUMLOCK", "NUMPAD_0", "NUMPAD_1", "NUMPAD_2", "NUMPAD_3", "NUMPAD_4", "NUMPAD_5", "NUMPAD_6", "NUMPAD_7", "NUMPAD_8", "NUMPAD_9", "PAUSE", "PERIOD", "PRIOR (PG UP)", "RBRACKET", "RCONTROL", "RETURN", "RIGHT", "R ALT", "RSHIFT", "RWIN", "SCROLL", "SEMICOLON", "SLASH", "SPACE", "SUBTRACT", "TAB", "UP", "ENTER (num pad)", "' (quote)"] ("keys pressed")
                        }
                      }
                      n246 = Insert Into Array(array=w286, index=w288, new element=w289) -> (w287:T1)
                    }
                    n247 = Wait (ms)(milliseconds to wait=u32 10) -> ()  [unwired: 1 out]
                    n248 = local read "seg"() -> (w275:bool)
                    n249 = local read "ambos"() -> (w276:bool)
                    n250 = local read "inver"() -> (w274:bool)
                    n251 = And(x=w276, y=w275) -> (x .and. y?=w273:bool)
                    n252 = Or(x=w274, y=w273) -> (x .or. y?=w272:bool)
                    n253 = case shown="False" w272 {
                      tunnel: [w283 w285] -> w278
                      tunnel: w277 -> [w283 w284]
                      frame False {
                      }
                      frame True {
                        n254 = Reverse 1D Array(array=w284) -> (reversed array=w285:T1)
                      }
                    }
                    "array2" <- w278
                  }
                  frame #3 {
                    n255 = property on="Comece" class="Str"("Visible"=TRUE) -> ()  [unwired: 2 in, 2 out]
                    n256 = Wait (ms)(milliseconds to wait="comece") -> ()  [unwired: 1 out]
                  }
                  frame #4 {
                    n257 = local read "size"() -> (w305:i32)
                    n258 = property on="Comece" class="Str"("Visible"=FALSE) -> ()  [unwired: 2 in, 2 out]
                    n259 = for {
                      N: w305 -> [_]
                      i -> [w310]
                      n260 = feedback #1() -> (w309:i32[])
                      n261 = call <vilib>:"Intialize Keyboard.vi"() -> ("device ID"=w312:refnum<k1>)  [unwired: 10 in, 1 out]
                      n262 = node-c288(i64 5 ("Period")) -> (w314:T2)  [unwired: 4 in]
                      n263 = feedback #2() -> (w308:dbl[])
                      n264 = timed-loop {
                        tunnel: w312 -> [w336]
                        timing: w314 -> [_]
                        timing-out: [_] -> w313
                        tunnel: w310 -> [w321]
                        tunnel: [w323] -> w306
                        tunnel: w309 -> [w322]
                        tunnel: [w319] -> w307
                        tunnel: w308 -> [w318]
                        i -> [w334]
                        stop <- w324 stop-if-true
                        n265 = node-c288() -> ()  [unwired: 1 in, 1 out]
                        n266 = local read "array2"() -> (w329:T1)
                        n267 = call-poly <vilib>:"Acquire Input Data.vi"("device ID"=w336) -> ("keys pressed"=w332:T1)  [unwired: 16 in, 2 out]
                        n268 = Multiply(x=5 ("y"), y=w334) -> (x*y=w317:i32)
                        n269 = Insert Into Array(array=w322, index=w321, new element=w317) -> (w323:i32[])
                        n270 = Index Array(array=w329, index=w321) -> (element=w316:T5)
                        n271 = Not Equal?(x=w332, y=w316) -> (x != y?=w330:bool[])
                        n272 = Equal?(x=w332, y=w316) -> (x = y?=w335:bool[])
                        n273 = Or Array Elements(Boolean array=w335) -> (logical OR=w331:bool)
                        n274 = Or Array Elements(Boolean array=w330) -> (logical OR=w328:bool)
                        n275 = Greater?(x=w317, y="sensib") -> (0:w326:bool)
                        n276 = Or(x=w328, y=w331) -> (x .or. y?=w325:bool)
                        n277 = And(x=w325, y=w326) -> (x .and. y?=w324:bool)
                        n278 = And(x=w326, y=w328) -> (x .and. y?=w327:bool)
                        n279 = case shown="True" w327 {
                          tunnel: [0.0 ("Erro_N1") 1.0 ("Erro_N1")] -> w320
                          frame False {
                          }
                          frame True {
                          }
                        }
                        n280 = Insert Into Array(array=w318, index=w321, new element=w320) -> (w319:dbl[])
                        n281 = node-c288() -> ()  [unwired: 1 in, 1 out]
                      }
                      "time" <- w306
                      "error" <- w307
                      n282 = feedback-in #1(w306) -> ()
                      n283 = feedback-in #2(w307) -> ()
                      n284 = node-c288(w313) -> ()  [unwired: 1 out]
                    }
                  }
                  frame #5 {
                    n285 = local read "error"() -> (w352:dbl[])
                    n286 = local read "size"() -> (w353:i32)
                    n287 = local read "size"() -> (w360:i32)
                    n288 = property on="Aguarde" class="Str"("Visible"=TRUE) -> ()  [unwired: 2 in, 2 out]
                    n289 = local read "time"() -> (w361:i32[])
                    n290 = Wait (ms)(milliseconds to wait="aguarde") -> ()  [unwired: 1 out]
                    n291 = Split 1D Array(array=w352, index=w353) -> (first subarray=w354:dbl[])  [unwired: 1 out]
                    n292 = local read "size"() -> (w345:i32)
                    n293 = Split 1D Array(array=w361, index=w360) -> (first subarray=w359:i32[])  [unwired: 1 out]
                    n294 = for {
                      N: w345 -> [_]
                      i -> [w367]
                      n295 = local read "time"() -> (w373:i32[])
                      n296 = local read "size"() -> (w374:i32)
                      n297 = Index Array(array=w373, index=w367) -> (element=w369:i32)
                      n298 = Split 1D Array(array=w373, index=w374) -> (first subarray=w372:i32[])  [unwired: 1 out]
                      n299 = Add Array Elements(numeric array=w372) -> (sum=w371:i32)
                      n300 = Multiply(x=0.01, y=w371) -> (x*y=w368:dbl)
                      n301 = Divide(x=w369, y=w368) -> (x/y=w365:dbl)
                      n302 = feedback #3() -> (w364:dbl[])
                      n303 = Insert Into Array(array=w364, index=w367, new element=w365) -> (w366:dbl[])
                      "tempo_rel" <- w366
                      n304 = feedback-in #3(w366) -> ()
                    }
                    n305 = Add Array Elements(numeric array=w354) -> (sum=w348:dbl)
                    n306 = Greater Or Equal?(x=w348, y=1.0) -> (x >= y?=w346:bool)
                    n307 = Add Array Elements(numeric array=w359) -> (sum=w358:i32)
                    n308 = case shown="True" w346 {
                      frame False {
                      }
                      frame True {
                        n309 = feedback #4() -> (w376:dbl)
                        n310 = Increment(x=w376) -> (x+1=w375:dbl)
                        n311 = feedback-in #4(w375) -> ()
                        n312 = local write "cont_erro"(w376) -> ()
                      }
                    }
                    n313 = feedback #5() -> (w350:dbl[])
                    n314 = Insert Into Array(array=w350, index=0, new element=w348) -> (w351:dbl[])
                    "erro" <- w351
                    n315 = feedback-in #5(w351) -> ()
                    n316 = feedback #6() -> (w355:i32[])
                    n317 = Insert Into Array(array=w355, index=0, new element=w358) -> (w356:i32[])
                    "total" <- w356
                    n318 = feedback-in #6(w356) -> ()
                  }
                }
              }
            }
          }
        }
        "cont_erro" <- 0.0 ("cont_erro")
      }
      frame #2 {
        n319 = flat-sequence {
          frame #0 {
            n320 = local read "total"() -> (w411:dbl[])
            n321 = call "Get User Input.vi"() -> ("string"=w425:string[])  [unwired: 10 in, 1 out]
            n322 = call-poly <vilib>:"Write To Spreadsheet File.vi"("format (%s)"="%s" ("format (%.3f)"), "1D data"=w425) -> ("new file path (Not A Path if cancelled)"=w424:path)  [unwired: 6 in]
            n323 = Reverse 1D Array(array=w411) -> (reversed array=w410:dbl[])
            n324 = Number To Decimal String(number=w410) -> (decimal integer string=w423:string[])  [unwired: 1 in]
            n325 = local read "erro"() -> (w385:dbl[])
            n326 = Build Array (concatenate)("Tempo", w423) -> (w427:string[])
            n327 = call-poly <vilib>:"Write To Spreadsheet File.vi"("delimiter (\\t)"=";" ("delimiter (\\t)"), "append to file? (new file:F)"=TRUE, "1D data"=w427, "file path (dialog if empty)"=w424) -> ("new file path (Not A Path if cancelled)"=w418:path)  [unwired: 4 in]
            n328 = Reverse 1D Array(array=w385) -> (reversed array=w409:dbl[])
            n329 = Number To Decimal String(number=w409) -> (decimal integer string=w419:string[])  [unwired: 1 in]
            n330 = Build Array (concatenate)("erros", w419) -> (w420:string[])
            n331 = local read "time"() -> (w386:i32[])
            n332 = call-poly <vilib>:"Write To Spreadsheet File.vi"("delimiter (\\t)"=";" ("delimiter (\\t)"), "append to file? (new file:F)"=TRUE, "1D data"=w420, "file path (dialog if empty)"=w418) -> ("new file path (Not A Path if cancelled)"=w403:path)  [unwired: 4 in]
            n333 = Reverse 1D Array(array=w386) -> (reversed array=w405:i32[])
            n334 = Number To Decimal String(number=w405) -> (decimal integer string=w406:string[])  [unwired: 1 in]
            n335 = local read "tempo_rel"() -> (w384:dbl[])
            n336 = Build Array (concatenate)("Tempo_abs_digito", w406) -> (w407:string[])
            n337 = call-poly <vilib>:"Write To Spreadsheet File.vi"("delimiter (\\t)"=";" ("delimiter (\\t)"), "append to file? (new file:F)"=TRUE, "1D data"=w407, "file path (dialog if empty)"=w403) -> ("new file path (Not A Path if cancelled)"=w388:path)  [unwired: 4 in]
            n338 = Reverse 1D Array(array=w384) -> (reversed array=w391:dbl[])
            n339 = Number To Decimal String(number=w391) -> (decimal integer string=w392:string[])  [unwired: 1 in]
            n340 = Build Array (concatenate)("Tempo_%_digito", w392) -> (w393:string[])
            n341 = local read "error"() -> (w383:dbl[])
            n342 = call-poly <vilib>:"Write To Spreadsheet File.vi"("delimiter (\\t)"=";" ("delimiter (\\t)"), "append to file? (new file:F)"=TRUE, "1D data"=w393, "file path (dialog if empty)"=w388) -> ("new file path (Not A Path if cancelled)"=w387:path)  [unwired: 4 in]
            n343 = local read "erro"() -> (w382:dbl[])
            n344 = Reverse 1D Array(array=w383) -> (reversed array=w398:dbl[])
            n345 = Array Size(array=w382) -> (size(s)=w381:i32)
            n346 = Number To Decimal String(number=w398) -> (decimal integer string=w399:string[])  [unwired: 1 in]
            n347 = Divide(x=w381, y=2) -> (x/y=w379:dbl)
            n348 = Build Array (concatenate)("erros_por_digito", w399) -> (w400:string[])
            n349 = Subtract(x=w379, y=1.0) -> (x-y=w377:dbl)
            n350 = Number To Decimal String(number=w377) -> (decimal integer string=w413:string)  [unwired: 1 in]
            n351 = Build Array("Spam", w413) -> (w414:string[])
            n352 = call-poly <vilib>:"Write To Spreadsheet File.vi"("delimiter (\\t)"=";" ("delimiter (\\t)"), "append to file? (new file:F)"=TRUE, "1D data"=w400, "file path (dialog if empty)"=w387) -> ("new file path (Not A Path if cancelled)"=w396:path)  [unwired: 4 in]
            n353 = call-poly <vilib>:"Write To Spreadsheet File.vi"("delimiter (\\t)"=";" ("delimiter (\\t)"), "append to file? (new file:F)"=TRUE, "1D data"=w414, "file path (dialog if empty)"=w396) -> ()  [unwired: 4 in, 1 out]
          }
        }
      }
    }
  }
